vi "Inline Wait.vi"(7 "Command":T1, 8 "error in (no error)":errorcluster, 10 "Dispatcher Interface in":refnum<class "Dispatcher Interface.lvclass">, 11 "Plugin Timing Group in":refnum<class "Scheduler Plugin Bundle.lvclass">) -> (0 "error out":errorcluster, 2 "Dispatcher Interface out":refnum<class "Dispatcher Interface.lvclass">, 3 "Plugin Timing Group out":refnum<class "Scheduler Plugin Bundle.lvclass">)   [LabVIEW 2017, in "Scheduler Plugin Bundle.lvclass"]
uses:
  Scheduler/Scheduler Plugin Bundle.lvclass
  Scheduler/Scheduler Transfer Group Bundle.lvclass
  Interfaces/Dispatcher/Dispatcher Interface.lvclass
  Interfaces/Dispatcher/Command.ctl
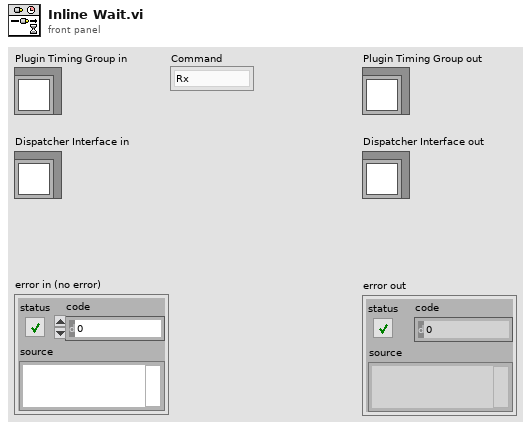
[diagram p1: front panel]
types:
  T1 = typedef "DSF Core.lvlib/Dispatcher Interface.lvclass/Command.ctl" = enum8{"Rx", "Tx", "Set Inline Buffer", "Shutdown"}
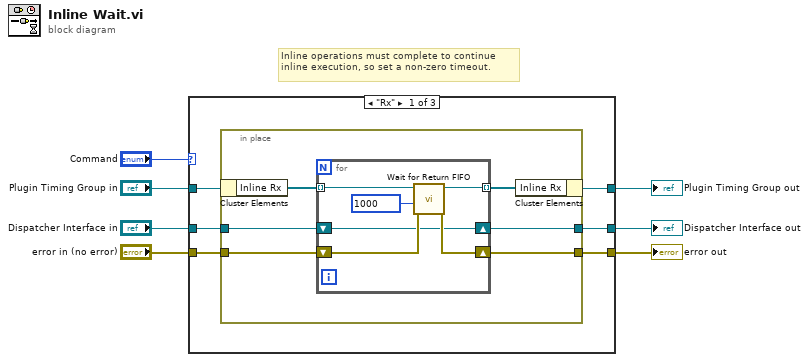
[diagram p0: block diagram]
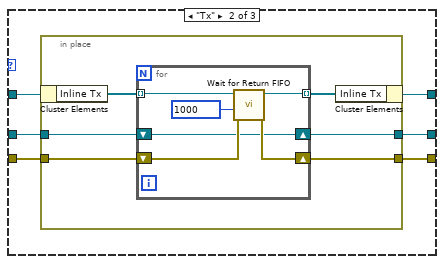
[diagram p2: hidden frame]
diagram:
  # "Inline operations must complete to continue inline execution, so set a non-zero timeout."
  n1 = case shown="\"Rx\"" "Command" {
    tunnel: [w13 w31 w46] -> w7
    tunnel: "Dispatcher Interface in" -> [w12 w30 w45]
    tunnel: [w11 w29 w45] -> w5
    tunnel: "error in (no error)" -> [w10 w28 w44]
    tunnel: [w9 w27 w44] -> w3
    tunnel: "Plugin Timing Group in" -> [w8 w26 w46]
    frame "Rx" {
      n2 = in-place {
        in-place-border: w12 -> [w17]
        in-place-border: [w16] -> w11
        in-place-border: [w15] -> w9
        in-place-border: w10 -> [w14]
        n3 = in-place-cluster #1(w8) -> ("Inline Rx"=w19:refnum<class "Scheduler Transfer Group Bundle.lvclass">[])
        n4 = for {
          tunnel: w19 -> [w25] mode=indexing
          tunnel: [w21] -> w18 mode=indexing
          shift-right: [w22] -> w16
          shift-left: w17 -> [w22]
          shift-right: [w23] -> w15
          shift-left: w14 -> [w24]
          n5 = call "Wait for Return FIFO.vi"("error in (no error)"=w24, "timeout (0 ms)"=1000, "Transfer Group Bundle in"=w25) -> ("error out"=w23:errorcluster, "Transfer Group Bundle out"=w21:refnum<class "Scheduler Transfer Group Bundle.lvclass">)  [unwired: 6 in, 1 out]
        }
        n6 = in-place-cluster #1("Inline Rx"=w18) -> (w13:refnum<class "Scheduler Plugin Bundle.lvclass">)
      }
    }
    frame "Tx" {
      n7 = in-place {
        in-place-border: w30 -> [w35]
        in-place-border: [w34] -> w29
        in-place-border: [w33] -> w27
        in-place-border: w28 -> [w32]
        n8 = in-place-cluster #2(w26) -> ("Inline Tx"=w37:refnum<class "Scheduler Transfer Group Bundle.lvclass">[])
        n9 = for {
          tunnel: w37 -> [w43] mode=indexing
          tunnel: [w39] -> w36 mode=indexing
          shift-right: [w40] -> w34
          shift-left: w35 -> [w40]
          shift-right: [w41] -> w33
          shift-left: w32 -> [w42]
          n10 = call "Wait for Return FIFO.vi"("error in (no error)"=w42, "timeout (0 ms)"=1000, "Transfer Group Bundle in"=w43) -> ("error out"=w41:errorcluster, "Transfer Group Bundle out"=w39:refnum<class "Scheduler Transfer Group Bundle.lvclass">)  [unwired: 6 in, 1 out]
        }
        n11 = in-place-cluster #2("Inline Tx"=w36) -> (w31:refnum<class "Scheduler Plugin Bundle.lvclass">)
      }
    }
    frame "Shutdown", Default {
    }
  }
  "Plugin Timing Group out" <- w7
  "Dispatcher Interface out" <- w5
  "error out" <- w3
